vi "9234_Update Channel List.vi"(10 "Channels":i32[](array[numeric]), 11 "MCListbox Refnum":refnum<vi>) -> ()   [LabVIEW 2020, in "Modules.lvlib" / "9234.lvclass"]
uses:
  9234.lvclass
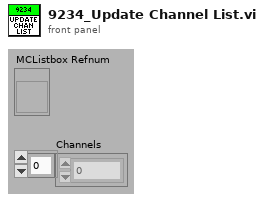
[diagram p1: front panel]
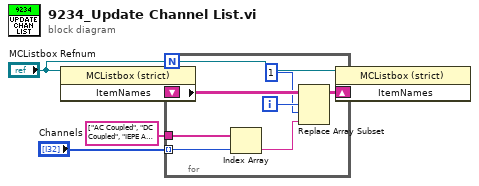
[diagram p0: block diagram]
diagram:
  n1 = property on="Property Node" class="MCListbox (strict)"(reference="MCListbox Refnum") -> ("ItemNames"=w2:string[][])  [unwired: 1 in, 2 out]
  n2 = for {
    shift-right: [w7] -> w4
    shift-left: w2 -> [w12]
    tunnel: string[] ["AC Coupled", "DC Coupled", "IEPE AC Coupled"] -> [w9]
    tunnel: "Channels" -> [w6] mode=indexing
    i -> [w11]
    n3 = Index Array(array=w9, index=w6) -> (element=w8:string)
    n4 = Replace Array Subset(array=w12, new element=w8, index (row)=w11, index (col)=1 ("disabled index (col)")) -> (w7:string[][])
  }
  n5 = property on="Property Node" class="MCListbox (strict)"(reference="MCListbox Refnum", "ItemNames"=w4) -> ()  [unwired: 1 in, 2 out]
